vi "B_2.vi"() -> ()   [LabVIEW 2020]
uses:
  <vilib>/numeric/Random Number (Range) DBL.vi
panel:
  out "Array Output":dbl[](array[numeric])
  out "Array Input":dbl[](array[numeric])
  in  "Numeric":i32
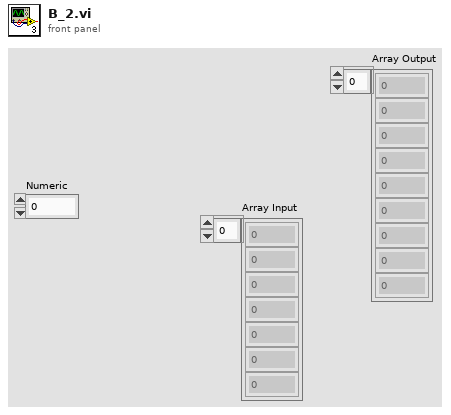
[diagram p1: front panel]
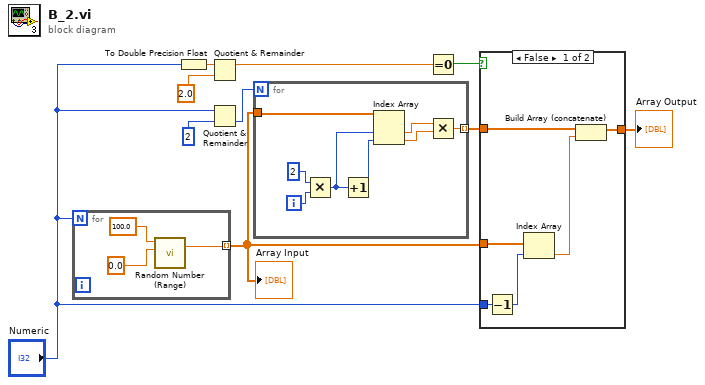
[diagram p0: block diagram]
diagram:
  n1 = for {
    N: "Numeric" -> [_]
    tunnel: [w11] -> w5 mode=indexing
    n2 = call-poly <vilib>:"Random Number (Range).vi"("lower bound (0)"=0.0, "upper bound (100)"=100.0) -> ("number"=w11:dbl)  [unwired: 9 in]
  }
  "Array Input" <- w5
  n3 = To Double Precision Float(number="Numeric") -> (double precision float=w1:dbl)
  n4 = Quotient & Remainder(x=w1, y=2.0) -> (x-y*floor(x/y)=w9:dbl)  [unwired: 1 out]
  n5 = Quotient & Remainder(x="Numeric", y=2) -> (floor(x/y)=w3:i32)  [unwired: 1 out]
  n6 = for {
    N: w3 -> [_]
    tunnel: [w18] -> w7 mode=indexing
    tunnel: w5 -> [w16]
    i -> [w17]
    n7 = Multiply(x=2, y=w17) -> (x*y=w15:i32)
    n8 = Increment(x=w15) -> (x+1=w14:i32)
    n9 = Index Array(array=w16, index #1=w15, index #2=w14) -> (element #1=w20:dbl, element #2=w19:dbl)
    n10 = Multiply(x=w20, y=w19) -> (x*y=w18:dbl)
  }
  n11 = Equal To 0?(x=w9) -> (x = 0?=w8:bool)
  n12 = case shown="False" w8 {
    tunnel: w7 -> [w24 w28]
    tunnel: [w26 w28] -> w6
    tunnel: "Numeric" -> [w23 _]
    tunnel: w5 -> [w25 _]
    frame False {
      n13 = Decrement(x=w23) -> (x-1=w22:i32)
      n14 = Index Array(array=w25, index=w22) -> (element=w27:dbl)
      n15 = Build Array (concatenate)(w24, w27) -> (w26:dbl[])
    }
    frame True {
    }
  }
  "Array Output" <- w6
